vi "Decode IDN Query Response.vi"(8 "error in (no error)":errorcluster, 11 "*IDN? Result":string) -> (0 "error out":errorcluster, 1 "Siglent Found":bool, 3 "Series ID":u32, 5 "Instrument Information":T1)   [LabVIEW 2021, in "Siglent SDS 1000 2000 Series.lvlib"]
doc: "Decodes the response to the *IDN? query. Outputs an identifier for each class of Siglent Oscilloscopes and a boolean = TRUE if the scope is found to be a SIGLENT by virtue of having the substring SIGLENT\" within the *IDN? response."
uses:
  <instrlib>/Siglent SDS 1000 2000 Series/Siglent SDS 1000 2000 Series.lvlib
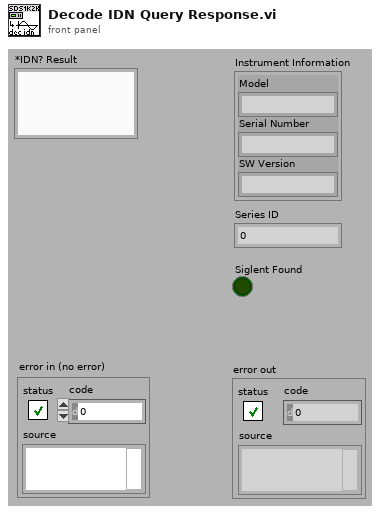
[diagram p1: front panel]
types:
  T1 = cluster{"Model":string, "Serial Number":string, "SW Version":string}
  T2 = cluster{"Status":bool, "Code":i32, "Source (VI Name)":string}
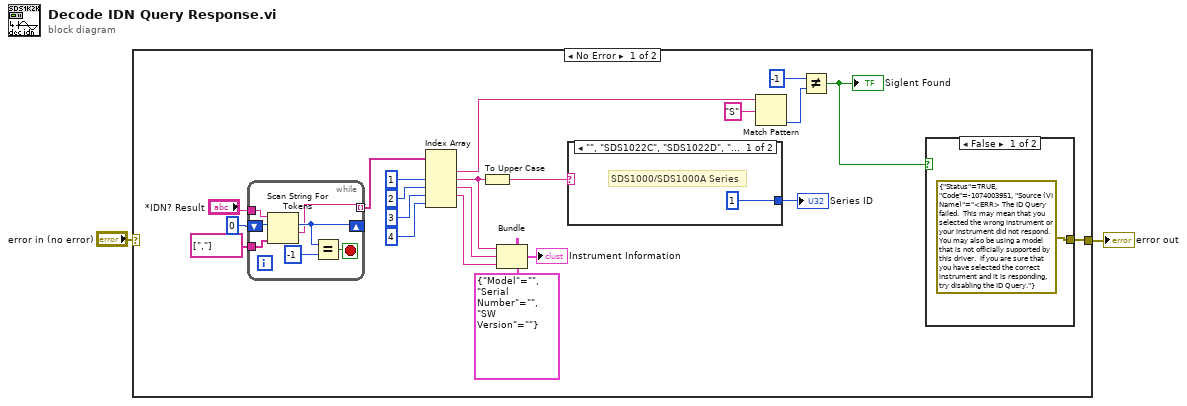
[diagram p0: block diagram]
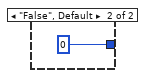
[diagram p3: hidden frame]
diagram:
  n1 = case shown="No Error" "error in (no error)" {
    selector: "error in (no error)" -> [_ w34]
    tunnel: [w4 w34] -> w1
    frame No Error {
      n2 = while {
        shift-right: [w29] -> _
        shift-left: 0 ("offset past token") -> [w31]
        tunnel: [w27] -> w17 mode=indexing
        tunnel: "*IDN? Result" -> [w26]
        tunnel: string[] [","] ("delimiters (\\s,\\t,\\r,\\n)") -> [w25]
        stop <- w30 stop-if-true
        n3 = Scan String For Tokens(6:w25, 8:w31, 9:w26) -> (1:w27:string, 2:w29:i32)  [unwired: 3 in, 2 out]
        n4 = Equal?(x=w29, y=-1) -> (x = y?=w30:bool)
      }
      n5 = Index Array(array=w17, index #2=1 ("index"), index #3=2 ("index"), index #4=3 ("index"), index #5=4 ("index")) -> (element #1=w16:string, element #2=w10:string, element #3=w9:string, element #4=w8:string)  [unwired: 1 in, 1 out]
      n6 = To Upper Case(1:w10) -> (0:w6:string)
      n7 = Bundle(cluster=T1 {"Model"="", "Serial Number"="", "SW Version"=""} ("Instrument Information"), "Model"=w10, "Serial Number"=w9, "SW Version"=w8) -> (→"Instrument Information":T1)
      n8 = case shown="\"\", \"SDS1022C\", \"SDS1022D\", \"SDS1022DL\", \"SDS1042C\", \"SDS1042D\", \"SDS1052A\", \"SDS1052DL\", \"SDS1062C\", \"SDS1062CM\", \"SDS1062D\", \"SDS1072A\", \"SDS1072CFL\", \"SDS1072CML\", \"SDS1072CNL\", \"SDS1074CFL\", \"SDS1102A\", \"SDS1102C\", \"SDS1102CFL\", \"SDS1102CM\", \"SDS1102CML\", \"SDS1102CN\", \"SDS1102CNL\", \"SDS1102D\", \"SDS1102DL\", \"SDS1104CFL\", \"SDS1152A\", \"SDS1152CM\", \"SDS1152CML\", \"SDS1202CFL\", \"SDS1202CN\", \"SDS1202CNL\", \"SDS1202D\", \"SDS1202DL\", \"SDS1204CFL\", \"SDS1302CFL\", \"SDS1304CFL\"" w6 {
        tunnel: [1 0] -> w5
        frame "", "SDS1022C", "SDS1022D", "SDS1022DL", "SDS1042C", "SDS1042D", "SDS1052A", "SDS1052DL", "SDS1062C", "SDS1062CM", "SDS1062D", "SDS1072A", "SDS1072CFL", "SDS1072CML", "SDS1072CNL", "SDS1074CFL", "SDS1102A", "SDS1102C", "SDS1102CFL", "SDS1102CM", "SDS1102CML", "SDS1102CN", "SDS1102CNL", "SDS1102D", "SDS1102DL", "SDS1104CFL", "SDS1152A", "SDS1152CM", "SDS1152CML", "SDS1202CFL", "SDS1202CN", "SDS1202CNL", "SDS1202D", "SDS1202DL", "SDS1204CFL", "SDS1302CFL", "SDS1304CFL" {
          # "SDS1000/SDS1000A Series"
        }
        frame "False", Default {
        }
      }
      "Series ID" <- w5
      n9 = Match Pattern(string=w16, regular expression="S") -> (offset past match=w22:i32)  [unwired: 1 in, 3 out]
      n10 = Not Equal?(x=-1, y=w22) -> (x != y?=w3:bool)
      "Siglent Found" <- w3
      n11 = case shown="False" w3 {
        tunnel: [T2 {"Status"=TRUE, "Code"=-1074003951, "Source (VI Name)"="<ERR> The ID Query failed.  This may mean that you selected the wrong instrument or your instrument did not respond.  You may also be using a model that is not officially supported by this driver.  If you are sure that you have selected the correct instrument and it is responding, try disabling the ID Query."} _] -> w4
        frame False {
        }
        frame True {
        }
      }
    }
    frame Error {
    }
  }
  "error out" <- w1
